vi "RecursiveDependenceies.vi"(8 "error in (no error)":errorcluster, 10 "Object":variant, 11 "JSON Schema in":string) -> (0 "error out":errorcluster, 3 "JSON Schema out":string)   [LabVIEW 2019, in "JSON-Schema.lvlib"]
uses:
  JSON-Schema.lvlib
  <vilib>/JDP Science/JSONtext/Next JSON Value.vi
  <vilib>/JDP Science/JSONtext/String Subset.vi
  <vilib>/JDP Science/JSONtext/Parsing/Advance past next JSON Value (inlined COPY).vi
  <vilib>/JDP Science/JSONtext/Parsing/Advance past whitespace.vi
  <vilib>/JDP Science/JSONtext/Parsing/Advance past String.vi
  <vilib>/JDP Science/JSONtext/Parsing/Advance past Number.vi
  <vilib>/JDP Science/JSONtext/Parsing/Advance past Line Ending.vi
  <vilib>/JDP Science/JSONtext/Parsing/Parse Full Path or Item Name.vi
  <vilib>/JDP Science/JSONtext/Parsing/Advance past Array.vi
  <vilib>/JDP Science/JSONtext/Parsing/Advance past Object.vi
  <vilib>/JDP Science/JSONtext/support/Error Cluster From Code.vi
  <vilib>/JDP Science/JSONtext/Offset/Find Item Locations by Path.vi
  <vilib>/JDP Science/JSONtext/JSONtext.lvlib
  <vilib>/Utility/Data Type/NI_Data Type.lvlib
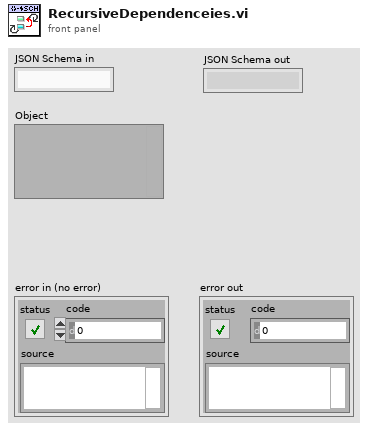
[diagram p1: front panel]
types:
  T1 = typedef "NI_Data Type.lvlib/Data Type.ctl" = enum8{"Invalid Type", "Void", "I8", "I16", "I32", "I64", "U8", "U16", "U32", "U64", "Single Float", "Double Float", "Extended Float", "Single Complex", "Double Complex", "Extended Complex", "Enum U8", "Enum U16", "Enum U32", "Enum U64", "Single Float With Unit", "Double Float With Unit", "Extended Float With Unit", "Single Complex with Unit", "Double Complex with Unit", "Extended Complex with Unit", "Boolean", "String", "Path", "Picture", "Tag", "Array", "Cluster", "Variant", "LV Variant", "Waveform", "Timestamp", "Digital Waveform", "Digital Data", "ExpressData", "Refnum", "External Data", "VI", "Poly VI", "LabVIEW Class Instance", "Fixed Point", "Set Collection", "Map Collection"}
  T2 = typedef "NI_Data Type.lvlib/Type Definition Info.ctl" = cluster{"Name":string, "Timestamp":u32}
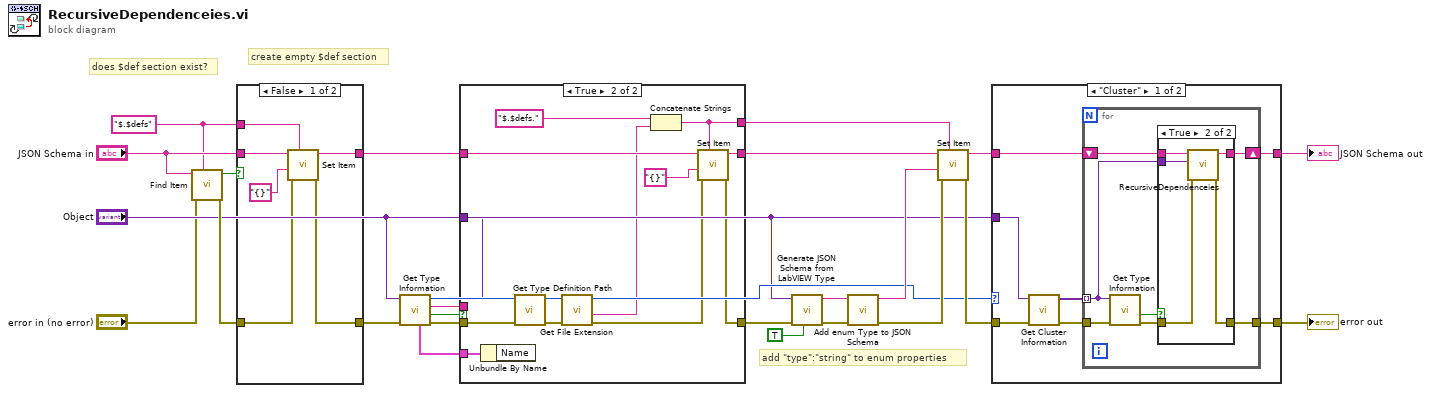
[diagram p0: block diagram]
diagram:
  w20 = "$.$defs" ("$Path or Item Name")
  # "add \"type\":\"string\" to enum properties"
  # "create empty $def section"
  # "does $def section exist?"
  n1 = call <vilib>:"Find Item.vi"("$Path or Item Name"=w20, "error in (no error)"="error in (no error)", "JSON"="JSON Schema in") -> ("error out"=w19:errorcluster, "Found"=w18:bool)  [unwired: 5 in, 2 out]
  n2 = case shown="False" w18 {
    tunnel: [w30 w32] -> w25
    tunnel: [w29 w33] -> w16
    tunnel: "JSON Schema in" -> [w28 w33]
    tunnel: w20 -> [w27 _]
    tunnel: w19 -> [w26 w32]
    frame False {
      n3 = call <vilib>:"Set Item.vi"("$Path or Item Name"=w27, "error in (no error)"=w26, "JSON to Insert"="{}", "JSON"=w28) -> ("error out"=w30:errorcluster, "<JSON>"=w29:string)  [unwired: 4 in, 1 out]
    }
    frame True {
    }
  }
  n4 = call <vilib>:"Get Type Information.vi"("error in (no error)"=w25, "variant"="Object") -> ("error out"=w23:errorcluster, "type definition"=w22:bool, "name"=w24:string, "type"=w4:T1, "type definition info"=w17:T2)  [unwired: 5 in]
  n5 = case shown="True" w22 {
    tunnel: w23 -> [w36 w38]
    tunnel: w24 -> [w34 _]
    tunnel: [w36 w44] -> w8
    tunnel: w17 -> [_ w49]
    tunnel: w16 -> [w35 w46]
    tunnel: [w35 w45] -> w5
    tunnel: [w34 w43] -> w6
    tunnel: "Object" -> [_ w40]
    frame False {
    }
    frame True {
      n6 = Unbundle By Name(w49) -> ()  [unwired: 1 out]
      n7 = call <vilib>:"Get Type Definition Path.vi"("error in (no error)"=w38, "variant"=w40) -> ("error out"=w41:errorcluster, "type definition path"=w42:path)  [unwired: 8 in]
      n8 = call <vilib>:"Get File Extension.vi"("error in (no error)"=w41, "file"=w42) -> ("error out"=w39:errorcluster, "filename without extension"=w37:string)  [unwired: 5 in, 3 out]
      n9 = Concatenate Strings("$.$defs." ("$Path or Item Name"), w37) -> (w43:string)
      n10 = call <vilib>:"Set Item.vi"("$Path or Item Name"=w43, "error in (no error)"=w39, "JSON to Insert"="{}", "JSON"=w46) -> ("error out"=w44:errorcluster, "<JSON>"=w45:string)  [unwired: 4 in, 1 out]
    }
  }
  n11 = call <vilib>:"Generate JSON Schema from LabVIEW Type.vi"("Strict Clusters"=TRUE, "error in (no error)"=w8, "Variant"="Object") -> ("error out"=w12:errorcluster, "JSON Schema"=w13:string)  [unwired: 7 in]
  n12 = call "Add enum Type to JSON Schema.vi"("error in (no error)"=w12, "JSON Schema in"=w13) -> ("error out"=w10:errorcluster, "JSON Schema out"=w11:string)  [unwired: 8 in]
  n13 = call <vilib>:"Set Item.vi"("$Path or Item Name"=w6, "error in (no error)"=w10, "JSON to Insert"=w11, "JSON"=w5) -> ("error out"=w7:errorcluster, "<JSON>"=w3:string)  [unwired: 4 in, 1 out]
  n14 = case shown="\"Cluster\"" w4 {
    tunnel: "Object" -> [w55 _]
    tunnel: w7 -> [w56 w72]
    tunnel: [w51 w72] -> w15
    tunnel: w3 -> [w54 w71]
    tunnel: [w50 w71] -> w14
    frame "Cluster" {
      n15 = call <vilib>:"Get Cluster Information.vi"("error in (no error)"=w56, "variant"=w55) -> ("error out"=w52:errorcluster, "cluster elements"=w53:variant[])  [unwired: 8 in]
      n16 = for {
        tunnel: w53 -> [w58] mode=indexing
        shift-right: [w62] -> w50
        shift-left: w54 -> [w63]
        tunnel: w52 -> [w59]
        tunnel: [w61] -> w51
        n17 = call <vilib>:"Get Type Information.vi"("error in (no error)"=w59, "variant"=w58) -> ("error out"=w60:errorcluster, "type definition"=w57:bool)  [unwired: 5 in, 3 out]
        n18 = case shown="True" w57 {
          tunnel: w63 -> [w64 w70]
          tunnel: [w64 w69] -> w62
          tunnel: [w65 w68] -> w61
          tunnel: w60 -> [w65 w67]
          tunnel: w58 -> [_ w66]
          frame False {
          }
          frame True {
            n19 = call "RecursiveDependenceies.vi"("error in (no error)"=w67, "Object"=w66, "JSON Schema in"=w70) -> ("error out"=w68:errorcluster, "JSON Schema out"=w69:string)  [unwired: 7 in]
          }
        }
      }
    }
    frame Default {
    }
  }
  "error out" <- w15
  "JSON Schema out" <- w14
